vi "OneTimeCalibSingle.vi"(8 "error in":errorcluster, 11 "MagSpecCamera in":refnum<class "MagSpecCamera.lvclass">) -> (0 "error out":errorcluster, 3 "MagSpecCamera in":refnum<class "MagSpecCamera.lvclass">)   [LabVIEW 2020, in "MagSpecCamera.lvclass"]
uses:
  MagSpecCamera.lvclass
  MagSpec_Bella/Controls/OneTimeCalculation.ctl
  shared/OnOffTypeDef.ctl
  MagSpecCamera.lvclass/MagSpecCamera.ctl
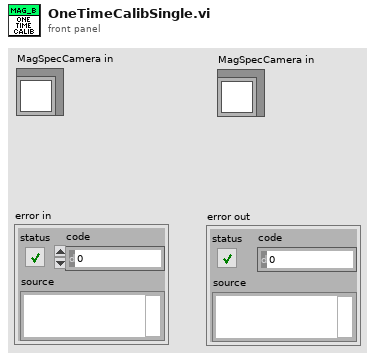
[diagram p1: front panel]
types:
  T1 = typedef "OneTimeCalculation.ctl" = cluster{"first Pixel pos [m]":dbl, "Pixel Size [mm]":dbl, "forward":T2}
  T2 = typedef "OnOffTypeDef.ctl" = enum16{"off", "on"}
  T3 = typedef "CameraSettings_File.ctl" = cluster{"FOV [mm]":dbl, "Left edge [mm]":dbl, "ROI Y offset":dbl, "ROI height":dbl, "ROI X offset":dbl, "ROI width":dbl, "Y center pixel":dbl, "Y Start":dbl, "Y End":dbl, "X Start":dbl, "X End":dbl, "rot [deg]":dbl}
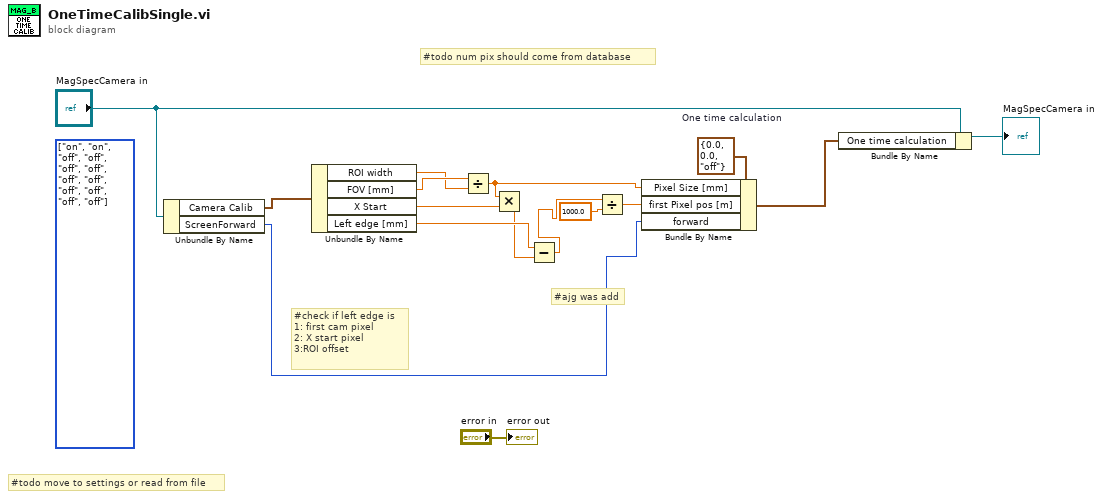
[diagram p0: block diagram]
diagram:
  w10 = T1 {"first Pixel pos [m]"=0.0, "Pixel Size [mm]"=0.0, "forward"=enum."off"}  # One time calculation
  (unwired) T2[] [enum."on", enum."on", enum."off", enum."off", enum."off", enum."off", enum."off", enum."off", enum."off", enum."off", enum."off", enum."off"] items=["off", "on"]
  # "#ajg was add"
  # "#todo num pix should come from database"
  # "#check if left edge is \n1: first cam pixel \n2: X start pixel\n3:ROI offset"
  # "#todo move to settings or read from file"
  n1 = Unbundle By Name("MagSpecCamera in") -> ("Camera Calib"=w13:T3, "ScreenForward"=w5:T2)
  n2 = Unbundle By Name(w13) -> ("ROI width"=w4:dbl, "FOV [mm]"=w11:dbl, "X Start"=w6:dbl, "Left edge [mm]"=w3:dbl)
  n3 = Divide(x=w11, y=w4) -> (x/y=w8:dbl)
  n4 = Multiply(x=w8, y=w6) -> (x*y=w2:dbl)
  n5 = Subtract(x=w3, y=w2) -> (x-y=w1:dbl)
  n6 = Divide(x=w1, y=1000.0) -> (x/y=w7:dbl)
  n7 = Bundle By Name(cluster=w10, "Pixel Size [mm]"=w8, "first Pixel pos [m]"=w7, "forward"=w5) -> (w15:T1)
  n8 = Bundle By Name(cluster="MagSpecCamera in", "One time calculation"=w15) -> (→"MagSpecCamera in":refnum<class "MagSpecCamera.lvclass">)
  "error out" <- "error in"
